vi "Read Joy Axis.vi"(8 "error in":errorcluster, 11 "TeleOp Data Cluster in":T1) -> (0 "error out":errorcluster, 3 "TeleOp Data Cluster out":T1)   [LabVIEW 2018]
uses:
  TypeDefs/Teleop Data Cluster.ctl
  TypeDefs/typedef_enum_Refnums.ctl
  TypeDefs/Joystick Axes.ctl
  <vilib>/Rock Robotics/WPI/Utilities/WPI_GetSetVariantRefNum.vi
panel:
  out "POVs":i16[](array[numeric])
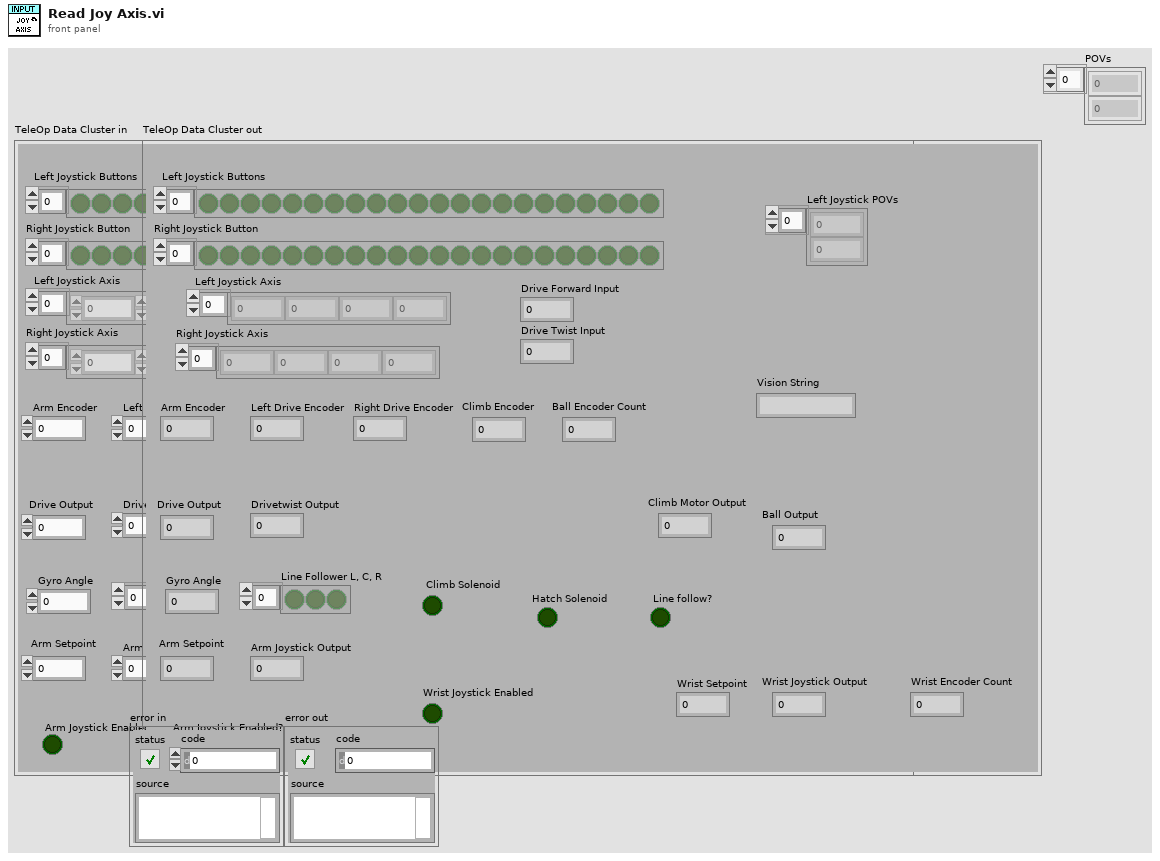
[diagram p1: front panel]
types:
  T1 = typedef "Teleop Data Cluster.ctl" = cluster{"Drive Forward Input ":dbl, "Drive Twist Input":dbl, "Drive Output":dbl, "Drivetwist Output":dbl, "Left Joystick Buttons":bool[], "Left Joystick Axis":dbl[], "Right Joystick Axis":dbl[], "Right Joystick Button":bool[], "Arm Encoder":dbl, "Left Drive Encoder":dbl, "Right Drive Encoder":dbl, "Gyro Angle ":dbl, "Arm Joystick Output  ":dbl, "Line Follower L, C, R ":bool[], "Line follow?":bool, " Climb Solenoid":bool, "Wrist Encoder Count":dbl, "Wrist Joystick Output":dbl, "Ball Encoder Count":dbl, "Ball Output":dbl, "Climb Encoder":dbl, "Climb Motor Output":dbl, " Hatch Solenoid":bool, "Arm Setpoint ":dbl, "Wrist Setpoint ":dbl, "Arm Joystick Enabled?":bool, "Wrist Joystick Enabled":bool, "Vision String":string, "Left Joystick POVs":i16[]}
  T2 = typedef "Joystick Axes.ctl" = enum16{"X Axis", "Y Axis", "Twist Axis", "Throttle"}
  T3 = typedef "typedef_enum_Refnums.ctl" = enum16{"Ball_Encoder", "Ball_Motor", "Camera", "Linefollow_3", "Linefollow_2", "Linefollow_1", "Gyro", "Hatch_Solenoid", "Climb_Back_Solenoid", "Arm_Encoder", "Arm_Motor", "Lift_Encoder", "Drive", "Drive_Motor_R", "Drive_Motor_L", "Drive_Encoder_R", "Drive_Encoder_L", "Joy_R", "Joy_L", "Wrist_Motor", "Wrist_Encoder", "Climb Upper Limit", "Climb Lower Limit ", "Climb_Front_Motor"}
  T4 = typedef "WPI_JoystickDevRef.ctl" = cluster{"Device":T5}
  T5 = typedef "WPI_JoystickDeviceEnum.ctl" = enum16{"USB 0", "USB 1", "USB 2", "USB 3", "USB 4", "USB 5"}
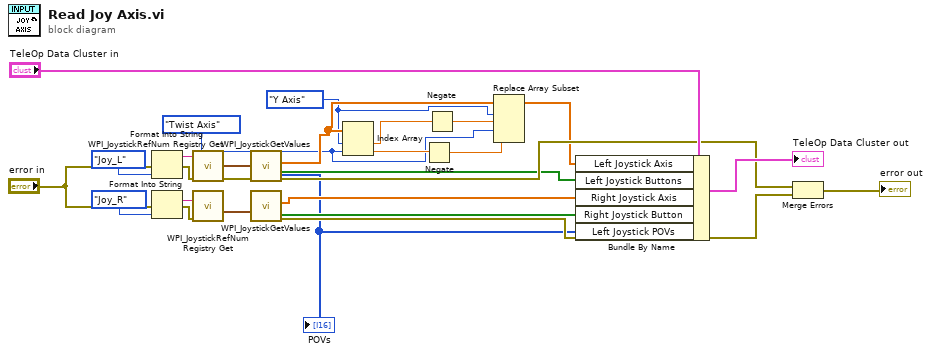
[diagram p0: block diagram]
diagram:
  w4 = Joystick_Axes."Twist Axis" ("Enum")
  w3 = Joystick_Axes."Y Axis" ("Enum")
  n1 = Format Into String(error in="error in", typedef_enum_Refnums."Joy_L" ("RefNums")) -> (resulting string=w27:string, error out=w18:errorcluster)  [unwired: 2 in]
  n2 = Format Into String(error in="error in", typedef_enum_Refnums."Joy_R" ("RefNums")) -> (resulting string=w24:string, error out=w14:errorcluster)  [unwired: 2 in]
  n3 = call <vilib>:"WPI_JoystickRefNum Registry Get.vi"("error in (no error)"=w18, "refnum name"=w27) -> ("error out"=w17:errorcluster, "JoystickDevRef"=w25:T4)  [unwired: 8 in]
  n4 = call <vilib>:"WPI_JoystickRefNum Registry Get.vi"("error in (no error)"=w14, "refnum name"=w24) -> ("JoystickDevRef"=w22:T4)  [unwired: 8 in, 1 out]
  n5 = call <vilib>:"WPI_JoystickGetValues.vi"("error in (no error)"=w17, "JoystickDevRef"=w25) -> ("error out"=w12:errorcluster, "Buttons"=w2:bool[], "Axes"=w8:dbl[], "POVs"=w1:i16[])  [unwired: 5 in, 1 out]
  "POVs" <- w1
  n6 = call <vilib>:"WPI_JoystickGetValues.vi"("JoystickDevRef"=w22) -> ("error out"=w13:errorcluster, "Buttons"=w21:bool[], "Axes"=w11:dbl[])  [unwired: 6 in, 2 out]
  n7 = Index Array(array=w8, index #1=w3, index #2=w4) -> (element #1=w10:dbl, element #2=w9:dbl)
  n8 = Negate(x=w9) -> (-x=w5:dbl)
  n9 = Negate(x=w10) -> (-x=w6:dbl)
  n10 = Replace Array Subset(array=w8, new element #1=w6, index #1=w3, new element #2=w5, index #2=w4) -> (w7:dbl[])
  n11 = Bundle By Name(cluster="TeleOp Data Cluster in", "Left Joystick Axis"=w7, "Left Joystick Buttons"=w2, "Right Joystick Axis"=w11, "Right Joystick Button"=w21, "Left Joystick POVs"=w1) -> (→"TeleOp Data Cluster out":T1)
  n12 = Merge Errors(w12, w13) -> (→"error out":errorcluster)
